vi "counter test.vi"() -> ()   [LabVIEW 2015]
panel:
  out "error out":errorcluster
  in  "Stop Button":bool
  out "data":dbl format="%0.2f"
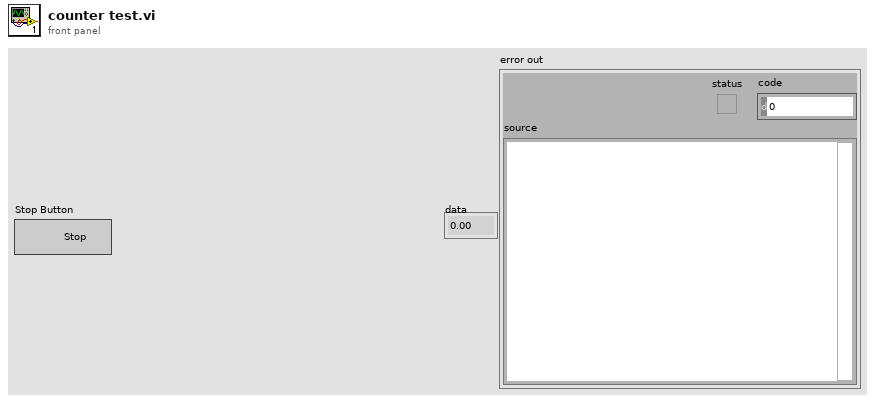
[diagram p1: front panel]
types:
  T1 = enum16{"init", "config", "start", "read", "stop"}
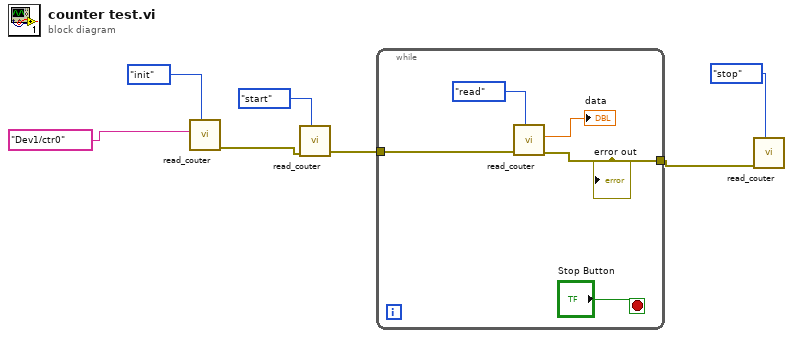
[diagram p0: block diagram]
diagram:
  n1 = call "read_couter.vi"("Enum"=T1."init", "counter"=tag "Dev1/ctr0") -> ("error out"=w3:errorcluster)  [unwired: 8 in, 1 out]
  n2 = call "read_couter.vi"("Enum"=T1."start", "error in"=w3) -> ("error out"=w2:errorcluster)  [unwired: 8 in, 1 out]
  n3 = while {
    tunnel: w2 -> [w12]
    tunnel: [w8] -> w5
    stop <- "Stop Button" stop-if-true
    n4 = call "read_couter.vi"("Enum"=T1."read", "error in"=w12) -> ("error out"=w8:errorcluster, "data"=→"data":dbl)  [unwired: 8 in]
    "error out" <- w8
  }
  n5 = call "read_couter.vi"("Enum"=T1."stop", "error in"=w5) -> ()  [unwired: 8 in, 2 out]
